vi "Test - Draw Lines 1.vi"() -> ()   [LabVIEW 2020, in "Raster.lvlib"]
uses:
  Raster.lvlib
  Point.ctl
  <vilib>/Utility/High Resolution Relative Seconds.vi
  Utility/Utility.lvlib
panel:
  out "Time [s]":dbl format="%.3p"
  in  "Numer Of Lines":i32
  out "new picture":picture
  # "(0,0)"
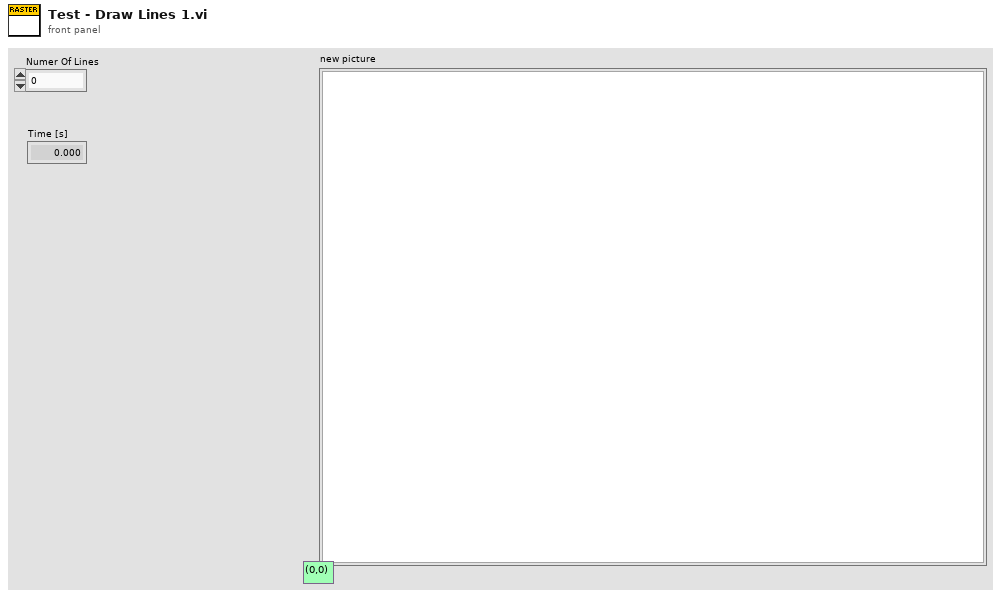
[diagram p1: front panel]
types:
  T1 = typedef "Raster.lvlib/Point.ctl" = cluster{"x":i32, "y":i32}
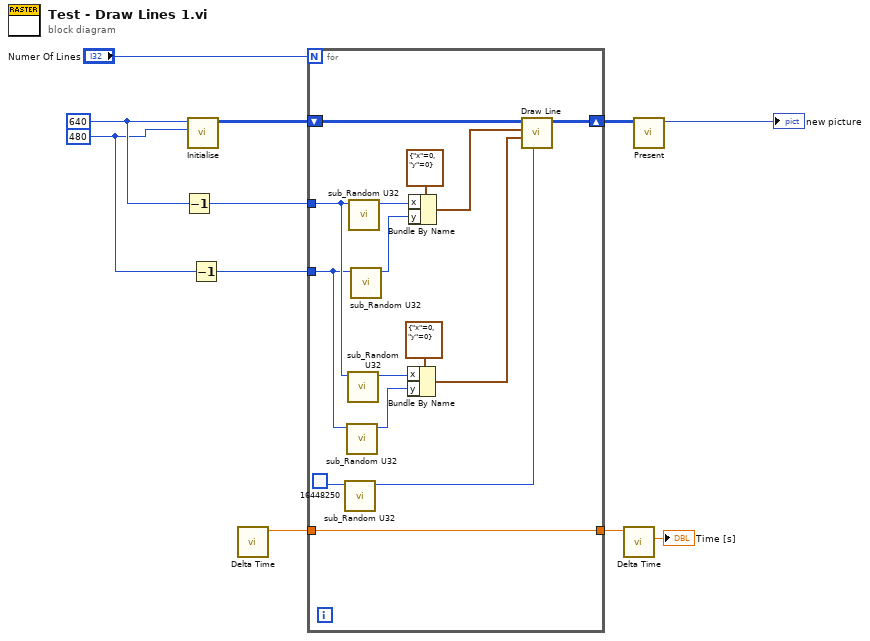
[diagram p0: block diagram]
diagram:
  w6 = u32 480 ("Screen Height")
  w7 = u32 640 ("Screen Width")
  n1 = Decrement(x=w7) -> (x-1=w5:u32)
  n2 = call "Initialise.vi"("Screen Height"=w6, "Screen Width"=w7) -> ("Pixel Data out"=w11:u32[][])  [unwired: 9 in]
  n3 = Decrement(x=w6) -> (x-1=w4:u32)
  n4 = call "Delta Time.vi"() -> ("Relative Seconds Out"=w3:dbl)  [unwired: 10 in, 1 out]
  n5 = for {
    N: "Numer Of Lines" -> [_]
    shift-right: [w25] -> w10
    shift-left: w11 -> [w26]
    tunnel: w5 -> [w17]
    tunnel: w4 -> [w16]
    tunnel: w3 -> [w14]
    tunnel: [w14] -> w2
    n6 = call <vilib>:"sub_Random U32.vi"("upper bound"=u32 16448250 ("Colour")) -> ("number"=w12:u32)  [unwired: 10 in]
    n7 = call <vilib>:"sub_Random U32.vi"("upper bound"=w16) -> ("number"=w20:u32)  [unwired: 10 in]
    n8 = call <vilib>:"sub_Random U32.vi"("upper bound"=w17) -> ("number"=w19:u32)  [unwired: 10 in]
    n9 = call <vilib>:"sub_Random U32.vi"("upper bound"=w17) -> ("number"=w22:u32)  [unwired: 10 in]
    n10 = call <vilib>:"sub_Random U32.vi"("upper bound"=w16) -> ("number"=w21:u32)  [unwired: 10 in]
    n11 = Bundle By Name(cluster=T1 {"x"=0, "y"=0} ("Point 1"), "x"=w19, "y"=w20) -> (w15:T1)
    n12 = Bundle By Name(cluster=T1 {"x"=0, "y"=0} ("Point 1"), "x"=w22, "y"=w21) -> (w23:T1)
    n13 = call "Draw Line.vi"("Colour"=w12, "Point 2"=w15, "Point 1"=w23, "Pixel Data in"=w26) -> ("Pixel Data out"=w25:u32[][])  [unwired: 7 in]
  }
  n14 = call "Delta Time.vi"("Relative Seconds In"=w2) -> ("Delta Seconds"=→"Time [s]":dbl)  [unwired: 9 in, 1 out]
  n15 = call "Present.vi"("Pixel Data in"=w10) -> ("2D Picture"=→"new picture":picture)  [unwired: 10 in]
